vi "MuxCardSwitch.vi"(6 "Single Needle":bool, 7 "Probe Card Channels":i32=32, 8 "error in (no error)":errorcluster, 9 "disabled channels":u32[](array[numeric]), 10 "Switch to channel":i32, 11 "Switching in":refnum<class "Switching.lvclass">) -> (0 "error out":errorcluster, 2 "last channel no.":i32, 3 "Switching out":refnum<class "Switching.lvclass">)   [LabVIEW 2018, in "Switching.lvclass"]
uses:
  Switching.lvclass
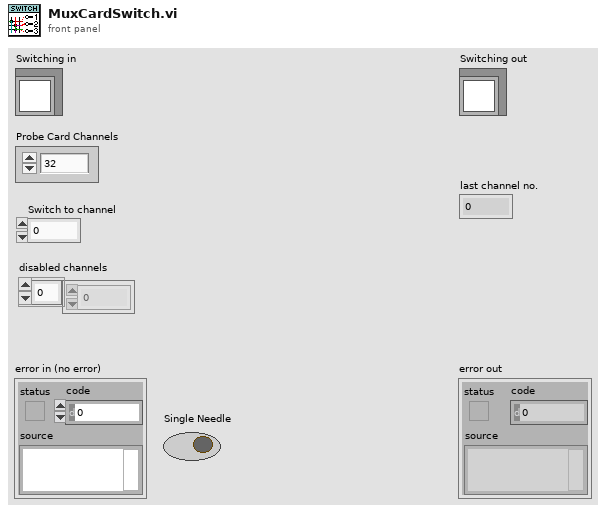
[diagram p1: front panel]
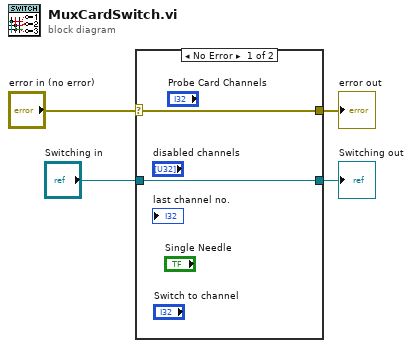
[diagram p0: block diagram]
diagram:
  n1 = case shown="No Error" "error in (no error)" {
    selector: "error in (no error)" -> [w5 w8]
    tunnel: [w5 w8] -> w3
    tunnel: [w6 w7] -> w1
    tunnel: "Switching in" -> [w6 w7]
    frame No Error {
    }
    frame Error {
    }
  }
  "error out" <- w3
  "Switching out" <- w1
